vi "Read Test Suite Result.vi"(11 "Test Suite In":refnum<class "LUnit Test Suite.lvclass">) -> (2 "Test Suite Result":refnum<class "Test Suite Result.lvclass">, 3 "Test Suite Out":refnum<class "LUnit Test Suite.lvclass">)   [LabVIEW 2020, in "LUnit Test Suite.lvclass"]
doc: "Read Test Suite Result. The Generate Test Suite vi needs to have been called before getting the result."
uses:
  LUnit Test Suite.lvclass
  Result Classes/Test Suite Result/Test Suite Result.lvclass
  LUnit Test Suite.lvclass/LUnit Test Suite.ctl
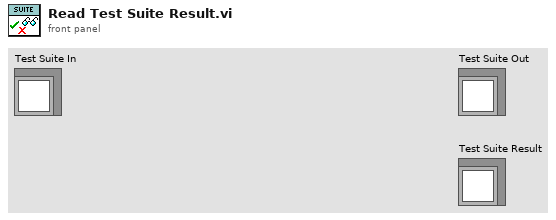
[diagram p1: front panel]
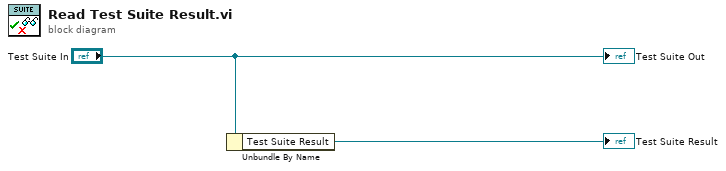
[diagram p0: block diagram]
diagram:
  n1 = Unbundle By Name("Test Suite In") -> ("Test Suite Result"=→"Test Suite Result":refnum<class "Test Suite Result.lvclass">)
  "Test Suite Out" <- "Test Suite In"
